vi "Wendy.vi"(6 "input":sgl[](array[numeric]), 8 "error in":errorcluster) -> (0 "error out":errorcluster)   [LabVIEW 2015]
uses:
  <vilib>/myRIO/Common/Instrument Driver Framework/myRIO v1.0/AudioOut Block/vis/myRIO v1.0 Close AudioOut Block.vi
  <vilib>/myRIO/Common/Instrument Driver Framework/myRIO v1.0/AudioOut Block/vis/myRIO v1.0 Unreserve AudioOut Block.vi
  <vilib>/myRIO/Common/Instrument Driver Framework/myRIO v1.0/Resource Manager/vis/myRIO v1.0 Shutdown Writing DMA.vi
  <vilib>/myRIO/Common/Instrument Driver Framework/myRIO v1.0/Resource Manager/vis/myRIO v1.0 Unreserve Channel List.vi
  <vilib>/myRIO/Common/Instrument Driver Framework/myRIO v1.0/AudioOut Block/vis/myRIO v1.0 Build MUX Configuration AudioOut Block.vi
  <vilib>/myRIO/Common/Instrument Driver Framework/myRIO v1.0/Resource Manager/vis/myRIO v1.0 Unreserve Channel.vi
  <vilib>/myRIO/Common/Instrument Driver Framework/myRIO v1.0/Resource Manager/vis/myRIO v1.0 Build Mutex Name.vi
  <vilib>/Utility/error.llb/Error Cluster From Error Code.vi
  <vilib>/myRIO/Common/Instrument Driver Framework/myRIO v1.0/AudioOut Block/vis/myRIO v1.0 AudioOut Block Write.vi
  <vilib>/myRIO/Common/Instrument Driver Framework/myRIO v1.0/Resource Manager/vis/myRIO v1.0 Block Write Resource Manager.vi
  <vilib>/myRIO/Common/Instrument Driver Framework/myRIO v1.0/Resource Manager/vis/myRIO v1.0 Block Write Counter.vi
  <vilib>/myRIO/Common/Instrument Driver Framework/Utilities/vis/Configuration Manager.vi
  <vilib>/myRIO/Common/Instrument Driver Framework/Utilities/vis/IO Manager.vi
  <vilib>/myRIO/Common/Instrument Driver Framework/myRIO v1.0/myRIO v1.0 Close.vi
  <vilib>/myRIO/Instrument Drivers/Onboard IO/AudioOut Block/AudioOut Block.lvlib
panel:
  # "(-1, 1)"
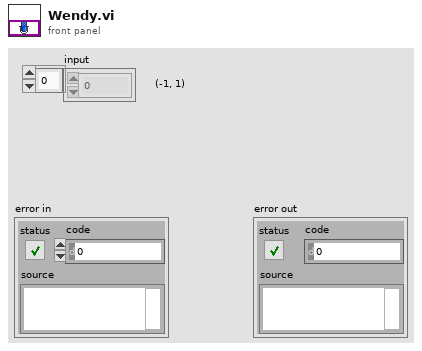
[diagram p1: front panel]
types:
  T1 = typedef "AudioOut Block.lvlib/AudioOut Block Reference.ctl" = cluster{"myRIO Reference":T2, "AudioOut (N Samples) Channels List":T6, "AudioOut (N Samples) Scaling Constants List":T8[]}
  T2 = typedef "myRIO Generic Hardware Reference.ctl" = cluster{"myRIO Model":T3, "myRIO Hardware Reference":T4}
  T3 = typedef "Hardware Version Enum.ctl" = enum16{"Unknown", "myRIO-1900", "myRIO-1950", "roboRIO"}
  T4 = typedef "myRIO v1.0 Reference.ctl" = cluster{"Generic FPGA Reference":T5, "Allow multiple opens":bool}
  T5 = typedef "Generic FPGA Reference.ctl" = refnum<k20>
  T6 = typedef "AudioOut Block Channels List.ctl" = T7[]
  T7 = typedef "AudioOut Block Channels Enum.ctl" = enum16{"Not Connected", "AudioOut/Left (N Samples)", "AudioOut/Right (N Samples)"}
  T8 = typedef "Analog Scaling Constants.ctl" = cluster{"LSB Weight (Volts)":dbl, "Offset (Volts)":dbl, "Signed?":bool}
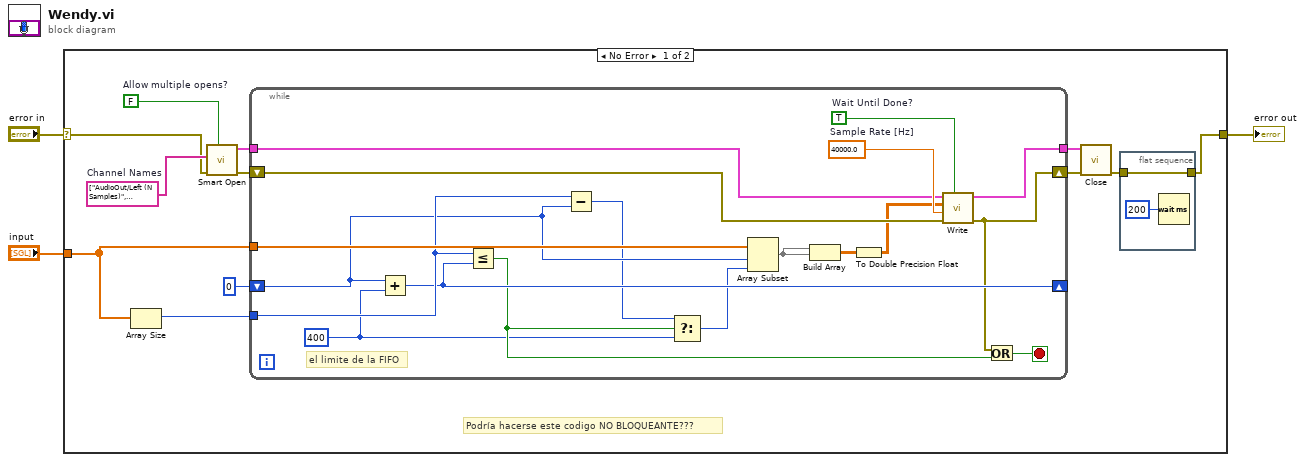
[diagram p0: block diagram]
diagram:
  n1 = case shown="No Error" "error in" {
    selector: "error in" -> [w8 w36]
    tunnel: "input" -> [w13 _]
    tunnel: [w4 w36] -> w2
    frame No Error {
      w12 = tag[] ["AudioOut/Left (N Samples)", "AudioOut/Right (N Samples)"]  # Channel Names
      w9 = FALSE  # Allow multiple opens?
      # "Podría hacerse este codigo NO BLOQUEANTE???"
      n2 = Array Size(array=w13) -> (size(s)=w15:i32)
      n3 = call <vilib>:"Smart Open.vi"("Allow multiple opens?"=w9, "error in (no error)"=w8, "Channel Names"=w12) -> ("error out"=w11:errorcluster, "AudioOut (N Samples) Ref Out"=w10:T1)  [unwired: 7 in]
      n4 = while {
        tunnel: w13 -> [w34]
        tunnel: w15 -> [w33]
        shift-right: [w31] -> _
        shift-left: 0 ("index") -> [w32]
        shift-right: [w21] -> w7
        shift-left: w11 -> [w20]
        tunnel: [w22] -> w6
        tunnel: w10 -> [w19]
        stop <- w35 stop-if-true
        w26 = TRUE  # Wait Until Done?
        w25 = 40000.0  # Sample Rate [Hz]
        w28 = 400 ("length")
        # "el limite de la FIFO"
        n5 = Add(x=w32, y=w28) -> (x+y=w31:i32)
        n6 = Less Or Equal?(x=w33, y=w31) -> (x <= y?=w30:bool)
        n7 = Subtract(x=w33, y=w32) -> (x-y=w27:i32)
        n8 = Select(t=w27, s=w30, f=w28) -> (s? t:f=w29:i32)
        n9 = Array Subset(array=w34, index=w32, length=w29) -> (w24:sgl[])
        n10 = Build Array(w24, w24) -> (w23:sgl[][])
        n11 = To Double Precision Float(number=w23) -> (double precision float=w18:dbl[][])
        n12 = call <vilib>:"Write.vi"("Wait Until Done?"=w26, "error in (no error)"=w20, "Sample Rate [Hz]"=w25, "Values"=w18, "AudioOut (N Samples) Ref In"=w19) -> ("error out"=w21:errorcluster, "AudioOut (N Samples) Ref Out"=w22:T1)  [unwired: 5 in]
        n13 = Or(x=w21, y=w30) -> (x .or. y?=w35:bool)
      }
      n14 = call <vilib>:"Close.vi"("error in (no error)"=w7, "AudioOut (N Samples) Ref In"=w6) -> ("error out"=w5:errorcluster)  [unwired: 9 in]
      n15 = flat-sequence {
        tunnel: w5 -> [w17]
        tunnel: [w17] -> w4
        frame #0 {
          n16 = Wait (ms)(milliseconds to wait=u32 200) -> ()  [unwired: 1 out]
        }
      }
    }
    frame Error {
    }
  }
  "error out" <- w2
